vi "SwerveDrive.vi"(8 "error in":errorcluster) -> ()   [LabVIEW 2019]
doc: "This VI runs in parallel to other tasks. It can contain as many user-defined periodic loops as you need. These can carry out PID or other sorts of timed response."
uses:
  <vilib>/Rock Robotics/WPI/ThirdParty/Phoenix-LabVIEW/Motor Controller/Controls/CTRE_Phoenix_MotorControl_ControlMode.ctl
  <vilib>/Rock Robotics/WPI/Utilities/WPI_GetSetVariantRefNum.vi
  <vilib>/Rock Robotics/Network Tables/NT Read Numeric Array.vi
  <vilib>/Rock Robotics/Network Tables/NT Write Numeric Array.vi
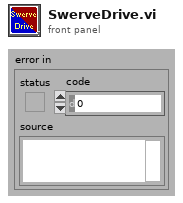
[diagram p1: front panel]
types:
  T1 = typedef "WPI_AnalogChannelDevRef.ctl" = cluster{"DevStatus":errorcluster, "Analog Channel":T2}
  T2 = typedef "FPGA_AIChannel.ctl" = enum8{"AI 0", "AI 1", "AI 2", "AI 3", "AI MXP 0", "AI MXP 1", "AI MXP 2", "AI MXP 3", "Invalid"}
  T3 = typedef "WPI_JoystickDevRef.ctl" = cluster{"Device":T4}
  T4 = typedef "WPI_JoystickDeviceEnum.ctl" = enum16{"USB 0", "USB 1", "USB 2", "USB 3", "USB 4", "USB 5"}
  T5 = typedef "WPI_MotorControlDeviceRef.ctl" = cluster{"DeviceStatus":errorcluster, "Type":T6, "PWM":cluster{"PWM Channel":T7, "DeadBand":T8}, "CAN":cluster{"Device Number":u8, "SetOutput VI Ref":variant, "GetOutput VI Ref":variant, "Enable VI Ref":variant, "Disable VI Ref":variant, "Data":variant}, "Invert":bool, "DIO PWM":cluster{"PWM \"Enable\" Channel":T7, "DIOChannel":T9, "PWM Rate":dbl}}
  T6 = typedef "WPI_MotorControlType.ctl" = enum16{"PWM", "CAN", "DIO PWM"}
  T7 = typedef "FPGA_DIOPWMChannel.ctl" = enum8{"PWM 0", "PWM 1", "PWM 2", "PWM 3", "PWM 4", "PWM 5", "PWM 6", "PWM 7", "PWM 8", "PWM 9", "PWM MXP 0", "PWM MXP 1", "PWM MXP 2", "PWM MXP 3", "PWM MXP 4", "PWM MXP 5", "PWM MXP 6", "PWM MXP 7", "PWM MXP 8", "PWM MXP 9", "Invalid"}
  T8 = typedef "WPI_PWMDeadband.ctl" = cluster{"Name":string, "maxPositivePwm":i32, "minPositivePwm":i32, "centerPwm":i32, "maxNegativePwm":i32, "minNegativePwm":i32, "angularRange":u16}
  T9 = typedef "FPGA_DIOChannel.ctl" = enum8{"DIO 0", "DIO 1", "DIO 2", "DIO 3", "DIO 4", "DIO 5", "DIO 6", "DIO 7", "DIO 8", "DIO 9", "DIO MXP 0", "DIO MXP 1", "DIO MXP 2", "DIO MXP 3", "DIO MXP 4", "DIO MXP 5", "DIO MXP 6", "DIO MXP 7", "DIO MXP 8", "DIO MXP 9", "DIO MXP 10", "DIO MXP 11", "DIO MXP 12", "DIO MXP 13", "DIO MXP 14", "DIO MXP 15", "SPI Port CS1", "SPI Port CS2", "SPI Port CS3", "SPI Port MISO", "SPI Port MOSI", "Invalid"}
  T10 = cluster{"PhoenixMotorControlDevRef":T5, "PhoenixMotorControlDevRef":T5, "PhoenixMotorControlDevRef":T5, "PhoenixMotorControlDevRef":T5}
  T11 = typedef "CTRE_Phoenix_MotorControl_ControlMode.ctl" = u16
  T12 = cluster{"Yaw":dbl, "Roll":dbl, "Pitch":dbl, "Heading":dbl, "Fused Heading":dbl}
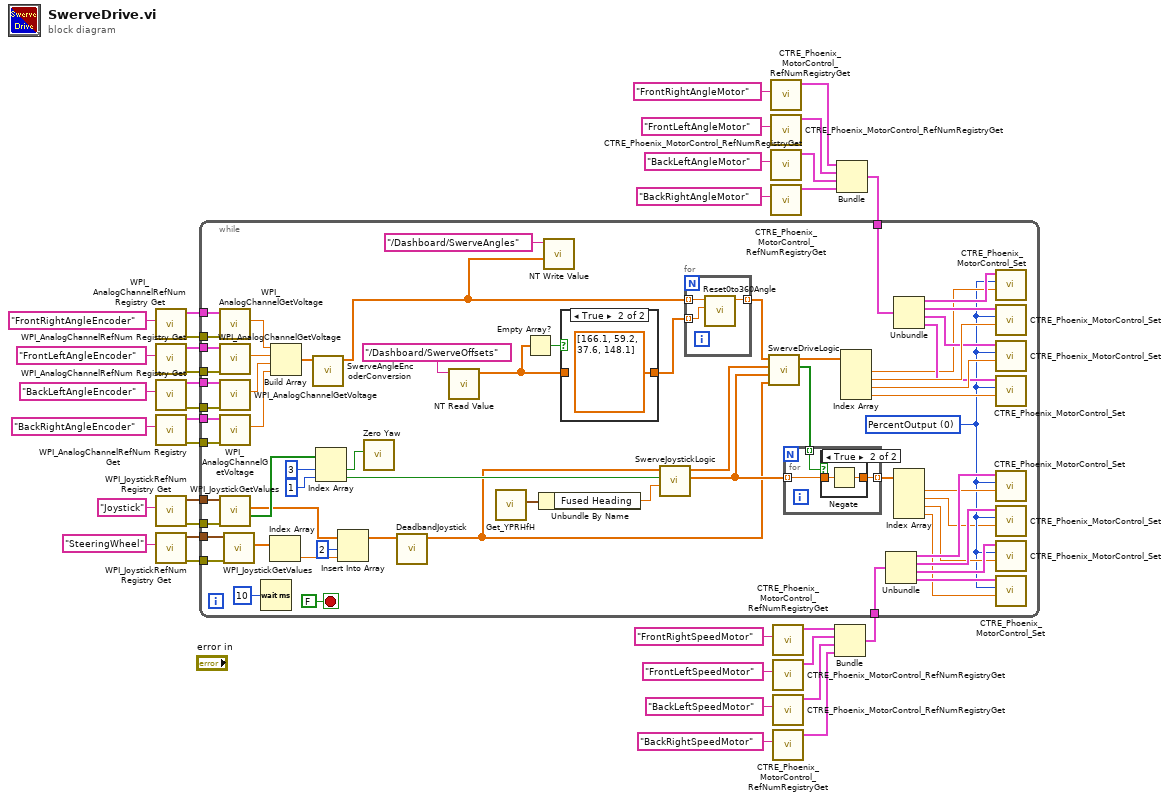
[diagram p0: block diagram]
diagram:
  n1 = call <vilib>:"WPI_AnalogChannelRefNum Registry Get.vi"("refnum name"="FrontRightAngleEncoder") -> ("error out"=w12:errorcluster, "AIDeviceRef"=w22:T1)  [unwired: 9 in]
  n2 = call <vilib>:"WPI_AnalogChannelRefNum Registry Get.vi"("refnum name"="FrontLeftAngleEncoder") -> ("error out"=w11:errorcluster, "AIDeviceRef"=w21:T1)  [unwired: 9 in]
  n3 = call <vilib>:"WPI_AnalogChannelRefNum Registry Get.vi"("refnum name"="BackLeftAngleEncoder") -> ("error out"=w10:errorcluster, "AIDeviceRef"=w20:T1)  [unwired: 9 in]
  n4 = call <vilib>:"WPI_AnalogChannelRefNum Registry Get.vi"("refnum name"="BackRightAngleEncoder") -> ("error out"=w9:errorcluster, "AIDeviceRef"=w19:T1)  [unwired: 9 in]
  n5 = call <vilib>:"WPI_JoystickRefNum Registry Get.vi"("refnum name"="Joystick") -> ("error out"=w4:errorcluster, "JoystickDevRef"=w5:T3)  [unwired: 1 in, 8 out]
  n6 = call <vilib>:"WPI_JoystickRefNum Registry Get.vi"("refnum name"="SteeringWheel") -> ("error out"=w2:errorcluster, "JoystickDevRef"=w3:T3)  [unwired: 1 in, 8 out]
  n7 = call <vilib>:"CTRE_Phoenix_MotorControl_RefNumRegistryGet.vi"("refnum name"="FrontRightAngleMotor") -> ("PhoenixMotorControlDevRef"=w13:T5)  [unwired: 9 in, 1 out]
  n8 = call <vilib>:"CTRE_Phoenix_MotorControl_RefNumRegistryGet.vi"("refnum name"="FrontLeftAngleMotor") -> ("PhoenixMotorControlDevRef"=w17:T5)  [unwired: 9 in, 1 out]
  n9 = call <vilib>:"CTRE_Phoenix_MotorControl_RefNumRegistryGet.vi"("refnum name"="BackLeftAngleMotor") -> ("PhoenixMotorControlDevRef"=w18:T5)  [unwired: 9 in, 1 out]
  n10 = call <vilib>:"CTRE_Phoenix_MotorControl_RefNumRegistryGet.vi"("refnum name"="BackRightAngleMotor") -> ("PhoenixMotorControlDevRef"=w15:T5)  [unwired: 9 in, 1 out]
  n11 = call <vilib>:"CTRE_Phoenix_MotorControl_RefNumRegistryGet.vi"("refnum name"="FrontRightSpeedMotor") -> ("PhoenixMotorControlDevRef"=w16:T5)  [unwired: 9 in, 1 out]
  n12 = call <vilib>:"CTRE_Phoenix_MotorControl_RefNumRegistryGet.vi"("refnum name"="FrontLeftSpeedMotor") -> ("PhoenixMotorControlDevRef"=w1:T5)  [unwired: 9 in, 1 out]
  n13 = call <vilib>:"CTRE_Phoenix_MotorControl_RefNumRegistryGet.vi"("refnum name"="BackLeftSpeedMotor") -> ("PhoenixMotorControlDevRef"=w23:T5)  [unwired: 9 in, 1 out]
  n14 = call <vilib>:"CTRE_Phoenix_MotorControl_RefNumRegistryGet.vi"("refnum name"="BackRightSpeedMotor") -> ("PhoenixMotorControlDevRef"=w24:T5)  [unwired: 9 in, 1 out]
  n15 = Bundle("PhoenixMotorControlDevRef"=w16, "PhoenixMotorControlDevRef"=w1, "PhoenixMotorControlDevRef"=w23, "PhoenixMotorControlDevRef"=w24) -> (w8:T10)  [unwired: 1 in]
  n16 = Bundle("PhoenixMotorControlDevRef"=w13, "PhoenixMotorControlDevRef"=w17, "PhoenixMotorControlDevRef"=w18, "PhoenixMotorControlDevRef"=w15) -> (w14:T10)  [unwired: 1 in]
  n17 = while {
    tunnel: w22 -> [w73]
    tunnel: w21 -> [w68]
    tunnel: w20 -> [w65]
    tunnel: w19 -> [w71]
    tunnel: w14 -> [w81]
    tunnel: w12 -> [w74]
    tunnel: w11 -> [w67]
    tunnel: w10 -> [w64]
    tunnel: w9 -> [w70]
    tunnel: w8 -> [w59]
    tunnel: w5 -> [w55]
    tunnel: w4 -> [w54]
    tunnel: w3 -> [w53]
    tunnel: w2 -> [w52]
    stop <- FALSE stop-if-true
    w75 = T11 0 items=["PercentOutput"=0, "Position"=1, "Velocity"=2, "Current"=3, "Follower"=5, "MotionProfile"=6, "MotionMagic"=7, "MotionProfileArc"=10, "Disabled"=15] ("Control Mode")
    n18 = call <vilib>:"WPI_AnalogChannelGetVoltage.vi"("error in (no error)"=w74, "AIDeviceRef"=w73) -> ("Voltage"=w72:dbl)  [unwired: 7 in, 2 out]
    n19 = call <vilib>:"WPI_AnalogChannelGetVoltage.vi"("error in (no error)"=w67, "AIDeviceRef"=w68) -> ("Voltage"=w66:dbl)  [unwired: 7 in, 2 out]
    n20 = call <vilib>:"WPI_AnalogChannelGetVoltage.vi"("error in (no error)"=w64, "AIDeviceRef"=w65) -> ("Voltage"=w63:dbl)  [unwired: 7 in, 2 out]
    n21 = call <vilib>:"WPI_AnalogChannelGetVoltage.vi"("error in (no error)"=w70, "AIDeviceRef"=w71) -> ("Voltage"=w69:dbl)  [unwired: 7 in, 2 out]
    n22 = call <vilib>:"WPI_JoystickGetValues.vi"("error in (no error)"=w54, "JoystickDevRef"=w55) -> ("Buttons"=w58:bool[], "Axes"=w42:dbl[])  [unwired: 5 in, 3 out]
    n23 = call <vilib>:"WPI_JoystickGetValues.vi"("error in (no error)"=w52, "JoystickDevRef"=w53) -> ("Axes"=w41:dbl[])  [unwired: 5 in, 4 out]
    n24 = Wait (ms)(milliseconds to wait=u32 10) -> ()  [unwired: 1 out]
    n25 = Index Array(array=w41) -> (element=w40:dbl)  [unwired: 1 in]
    n26 = Build Array(w72, w66, w63, w69) -> (w80:dbl[])
    n27 = call "SwerveAngleEncoderConversion.vi"("Voltages"=w80) -> ("Angles"=w46:dbl[])  [unwired: 10 in]
    n28 = Index Array(array=w58, index #1=3 ("index"), index #2=1 ("index")) -> (element #1=w43:bool, element #2=w44:bool)
    n29 = Insert Into Array(array=w42, index=2, new element=w40) -> (w38:dbl[])
    n30 = call <vilib>:"Zero Yaw.vi"("Zero"=w43) -> ()  [unwired: 11 in]
    n31 = call "DeadbandJoystick.vi"("InputArray"=w38) -> ("OutputArray"=w37:dbl[])  [unwired: 10 in]
    n32 = call-poly <vilib>:"NT Read Value.vi"("Name"="/Dashboard/SwerveOffsets") -> ("Numeric Array"=w51:dbl[])  [unwired: 9 in, 1 out]
    n33 = call <vilib>:"Get_YPRHfH.vi"() -> ("YRPHfH"=w60:T12)  [unwired: 11 in]
    n34 = Empty Array?(array=w51) -> (empty?=w50:bool)
    n35 = Unbundle By Name(w60) -> ("Fused Heading"=w45:dbl)
    n36 = call-poly <vilib>:"NT Write Value.vi"("Numeric Array"=w46, "Name"="/Dashboard/SwerveAngles") -> ()  [unwired: 9 in, 1 out]
    n37 = case shown="True" w50 {
      tunnel: [w100 dbl[] [166.1, 59.2, 37.6, 148.1] ("Numeric Array")] -> w49
      tunnel: w51 -> [w100 _]
      frame False {
      }
      frame True {
      }
    }
    n38 = call "SwerveJoystickLogic.vi"("Gyro"=w45, "TankMode"=w44, "Joystick Axes"=w37) -> ("Speeds"=w84:dbl[], "Angles"=w86:dbl[])  [unwired: 6 in]
    n39 = for {
      tunnel: w46 -> [w103] mode=indexing
      tunnel: [w104] -> w87 mode=indexing
      tunnel: w49 -> [w102] mode=indexing
      n40 = call "Reset0to360Angle.vi"("Offset"=w102, "AngleInput"=w103) -> ("AngleOutput"=w104:dbl)  [unwired: 9 in]
    }
    n41 = call "SwerveDriveLogic.vi"("Joystick Axes"=w37, "Speeds"=w84, "AngleSetpoints"=w86, "AngleEncoders"=w87) -> ("AngleMotorsReversed"=w88:bool[], "AngleMotorOutputs"=w85:dbl[])  [unwired: 6 in]
    n42 = for {
      tunnel: w84 -> [w106] mode=indexing
      tunnel: [w107] -> w93 mode=indexing
      tunnel: w88 -> [w105] mode=indexing
      n43 = case shown="True" w105 {
        tunnel: w106 -> [w108 w110]
        tunnel: [w108 w109] -> w107
        frame False {
        }
        frame True {
          n44 = Negate(x=w110) -> (-x=w109:dbl)
        }
      }
    }
    n45 = Index Array(array=w85) -> (element #1=w78:dbl, element #2=w98:dbl, element #3=w97:dbl, element #4=w79:dbl)  [unwired: 4 in]
    n46 = Unbundle(w59) -> ("PhoenixMotorControlDevRef"=w83:T5, "PhoenixMotorControlDevRef"=w92:T5, "PhoenixMotorControlDevRef"=w91:T5, "PhoenixMotorControlDevRef"=w90:T5)
    n47 = Unbundle(w81) -> ("PhoenixMotorControlDevRef"=w96:T5, "PhoenixMotorControlDevRef"=w95:T5, "PhoenixMotorControlDevRef"=w94:T5, "PhoenixMotorControlDevRef"=w89:T5)
    n48 = Index Array(array=w93) -> (element #1=w77:dbl, element #2=w61:dbl, element #3=w76:dbl, element #4=w62:dbl)  [unwired: 4 in]
    n49 = call <vilib>:"CTRE_Phoenix_MotorControl_Set.vi"("Output"=w78, "Control Mode"=w75, "PhoenixMotorControlDevRef"=w96) -> ()  [unwired: 7 in, 2 out]
    n50 = call <vilib>:"CTRE_Phoenix_MotorControl_Set.vi"("Output"=w98, "Control Mode"=w75, "PhoenixMotorControlDevRef"=w95) -> ()  [unwired: 7 in, 2 out]
    n51 = call <vilib>:"CTRE_Phoenix_MotorControl_Set.vi"("Output"=w97, "Control Mode"=w75, "PhoenixMotorControlDevRef"=w94) -> ()  [unwired: 7 in, 2 out]
    n52 = call <vilib>:"CTRE_Phoenix_MotorControl_Set.vi"("Output"=w79, "Control Mode"=w75, "PhoenixMotorControlDevRef"=w89) -> ()  [unwired: 7 in, 2 out]
    n53 = call <vilib>:"CTRE_Phoenix_MotorControl_Set.vi"("Output"=w77, "Control Mode"=w75, "PhoenixMotorControlDevRef"=w83) -> ()  [unwired: 7 in, 2 out]
    n54 = call <vilib>:"CTRE_Phoenix_MotorControl_Set.vi"("Output"=w61, "Control Mode"=w75, "PhoenixMotorControlDevRef"=w92) -> ()  [unwired: 7 in, 2 out]
    n55 = call <vilib>:"CTRE_Phoenix_MotorControl_Set.vi"("Output"=w76, "Control Mode"=w75, "PhoenixMotorControlDevRef"=w91) -> ()  [unwired: 7 in, 2 out]
    n56 = call <vilib>:"CTRE_Phoenix_MotorControl_Set.vi"("Output"=w62, "Control Mode"=w75, "PhoenixMotorControlDevRef"=w90) -> ()  [unwired: 7 in, 2 out]
  }
